vi "invernadero.vi"() -> ()   [LabVIEW 2016]
uses:
  <vilib>/Instr/_visa.llb/VISA Configure Serial Port (Instr).vi
panel:
  out "valor sensor luz":dbl
  out "Boolean 3":bool
  out "?":dbl(knob) scale=0.0..100.0
  out "Boolean 2":bool
  out "HUMEDAD RELATIVA (HR)":dbl(slide) scale=0.0..1000.0
  out "HUMEDAD RELATIVA (HR)":dbl(slide) scale=0.0..100.0
  out "Boolean":bool
  in  "ventilador 3":bool
  in  "ventilador 2":bool
  out "FAHRENHEIT °F":dbl(slide) scale=0.0..100.0
  out "CENTIGRADOS °C":dbl(slide) scale=0.0..70.0
  out "HR Actual":dbl
  in  "Ventana 2":bool
  in  "Ventana 1":bool
  in  "ventilador":bool
  out "Temperatura Actual":dbl
  out "temperatura Actual":dbl caption="temperatura Actual 2"
  in  "Detener":bool
  out "read buffer":string
  in  "PUERTO":refnum<visa-resource-name>
  out "HR Actual":dbl
  # "INVERNADERO"
  # "CONEXION"
  # "TEMPERATURA"
  # "HUMEDAD"
  # "TIEMPO"
  # "AIRE"
  # "SUELO"
  # "Noche"
  # "Dia"
  # "ILUMINACIÓN"
  # "Minima: 50 F\nMaxima: 68 F"
  # "Minima: 10 °C\nMaxima: 20 °C"
  # "Humedad Relativa Optima: entre 50 y 70%"
  # "VENTANAS"
  # "RIEGO"
  # "VENTILACION"
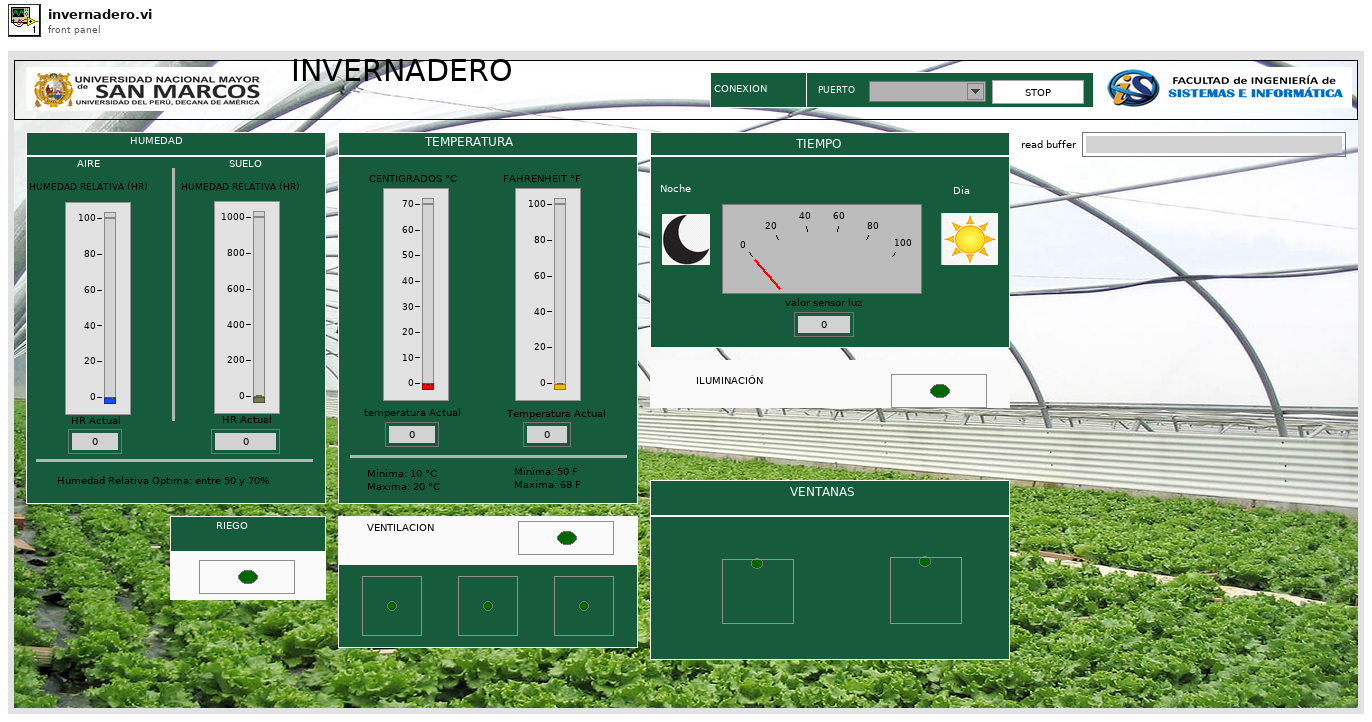
[diagram p1: front panel]
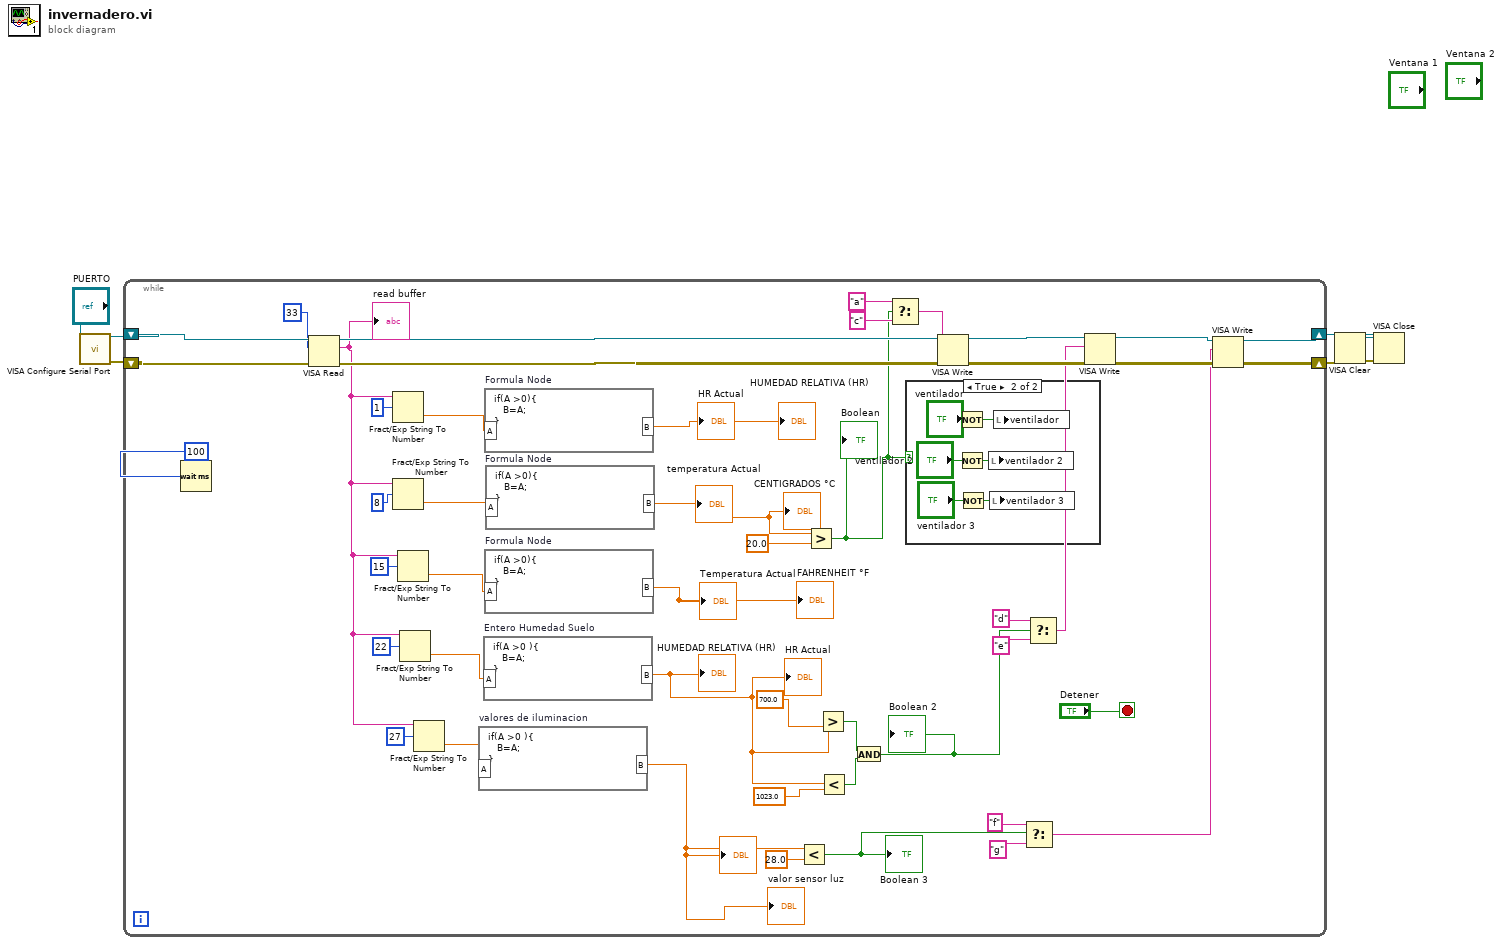
[diagram p0: block diagram]
diagram:
  n1 = call-poly "VISA Configure Serial Port"("VISA resource name"="PUERTO") -> ("VISA resource name out"=w5:refnum<visa-resource-name>, "error out"=w6:errorcluster)  [unwired: 13 in]
  n2 = while {
    shift-right: [w10] -> w3
    shift-left: w6 -> [w37]
    shift-right: [w11] -> w4
    shift-left: w5 -> [w38]
    stop <- "Detener" stop-if-true
    n3 = Wait (ms)(milliseconds to wait=u32 100) -> ()  [unwired: 1 out]
    n4 = VISA Read(VISA resource name=w38, byte count=u32 33, error in (no error)=w37) -> (VISA resource name out=w45:refnum<visa-resource-name>, read buffer=w18:string, error out=w44:errorcluster)  [unwired: 1 out]
    "read buffer" <- w18
    n5 = Fract/Exp String To Number(string=w18, offset=1) -> (number=w51:dbl)  [unwired: 2 in, 1 out]
    n6 = Fract/Exp String To Number(string=w18, offset=8) -> (number=w50:dbl)  [unwired: 2 in, 1 out]
    n7 = Fract/Exp String To Number(string=w18, offset=15) -> (number=w49:dbl)  [unwired: 2 in, 1 out]
    n8 = Fract/Exp String To Number(string=w18, offset=22) -> (number=w33:dbl)  [unwired: 2 in, 1 out]
    n9 = Fract/Exp String To Number(string=w18, offset=27) -> (number=w19:dbl)  [unwired: 2 in, 1 out]
    n10 = formula code="if(A >0 ){\n   B=A;\n}" "valores de iluminacion"("A"=w19) -> ("B"=w8:dbl)
    "?" <- w8
    "valor sensor luz" <- w8
    n11 = formula code="if(A >0 ){\n   B=A;\n}" "Entero Humedad Suelo"("A"=w33) -> ("B"=w23:dbl)
    "HUMEDAD RELATIVA (HR)" <- w23
    "HR Actual" <- w23
    n12 = formula code="if(A >0){\n   B=A;\n}"("A"=w51) -> ("B"=→"HR Actual" →"HUMEDAD RELATIVA (HR)":dbl)
    n13 = formula code="if(A >0){\n   B=A;\n}"("A"=w49) -> ("B"=→"Temperatura Actual" →"FAHRENHEIT °F":dbl)
    n14 = formula code="if(A >0){\n   B=A;\n}"("A"=w50) -> ("B"=w41:dbl)
    "temperatura Actual" <- w41
    "CENTIGRADOS °C" <- w41
    n15 = Less?(x=w8, y=28.0) -> (x < y?=w14:bool)
    "Boolean 3" <- w14
    n16 = Greater?(x=w41, y=20.0) -> (0:w30:bool)
    "Boolean" <- w30
    n17 = Greater?(x=w23, y=700.0) -> (0:w26:bool)
    n18 = Less?(x=w23, y=1023.0) -> (x < y?=w25:bool)
    n19 = And(x=w26, y=w25) -> (x .and. y?=w21:bool)
    "Boolean 2" <- w21
    n20 = Select(t="a", s=w30, f="c") -> (s? t:f=w46:string)
    n21 = case shown="True" w30 {
      frame False {
      }
      frame True {
        n22 = Not(x="ventilador") -> (.not. x?=w59:bool)
        n23 = Not(x="ventilador 2") -> (.not. x?=w58:bool)
        n24 = Not(x="ventilador 3") -> (.not. x?=w56:bool)
        n25 = local write "ventilador 2"(w58) -> ()
        n26 = local write "ventilador 3"(w56) -> ()
        n27 = local write "ventilador"(w59) -> ()
      }
    }
    n28 = VISA Write(VISA resource name=w45, write buffer=w46, error in (no error)=w44) -> (VISA resource name out=w32:refnum<visa-resource-name>, error out=w31:errorcluster)  [unwired: 1 out]
    n29 = Select(t="f", s=w14, f="g") -> (s? t:f=w9:string)
    n30 = Select(t="d", s=w21, f="e") -> (s? t:f=w27:string)
    n31 = VISA Write(VISA resource name=w32, write buffer=w27, error in (no error)=w31) -> (VISA resource name out=w13:refnum<visa-resource-name>, error out=w12:errorcluster)  [unwired: 1 out]
    n32 = VISA Write(VISA resource name=w13, write buffer=w9, error in (no error)=w12) -> (VISA resource name out=w11:refnum<visa-resource-name>, error out=w10:errorcluster)  [unwired: 1 out]
  }
  n33 = VISA Clear(VISA resource name=w4, error in (no error)=w3) -> (VISA resource name out=w2:refnum<visa-resource-name>, error out=w1:errorcluster)
  n34 = VISA Close(VISA resource name=w2, error in (no error)=w1) -> ()  [unwired: 1 out]
